vi "Edit Color List Dialog.vi"(10 "Color List":u32[](array[colorbox])=[16777225, 16448250, 16448250, 16448250, 16448250, 16448250, 16448250, 16448250, 16448250, 16448250], 11 "Color List Name":string) -> (0 "OK?":bool, 2 "Color List (out)":u32[](array[colorbox]), 3 "Color List Name (out)":string)   [LabVIEW 2021, in "Graphs.lvlib"]
uses:
  Graphs.lvlib
panel:
  in  "Cancel":bool
  in  "OK":bool
  out "# Colors":i32
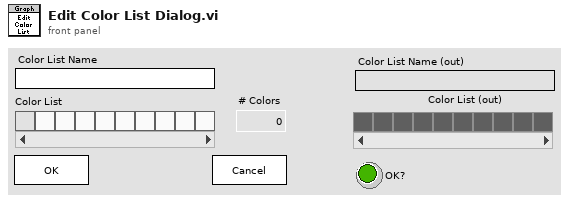
[diagram p1: front panel]
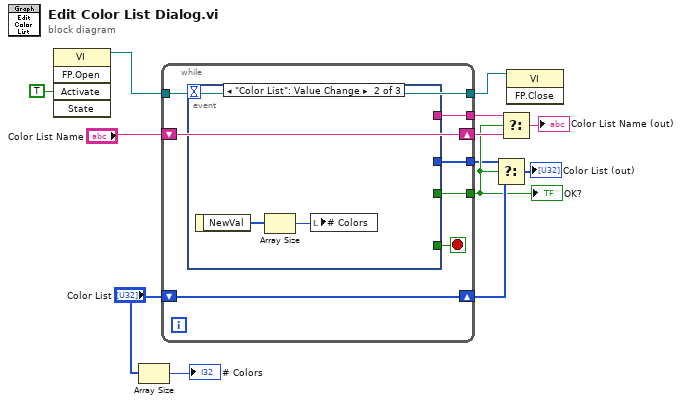
[diagram p0: block diagram]
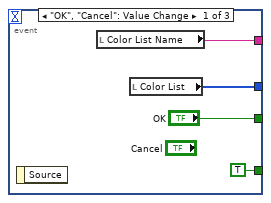
[diagram p2: hidden frame]
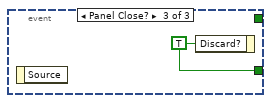
[diagram p3: hidden frame]
diagram:
  n1 = invoke class="VI" method="FP.Open"("Activate"=TRUE ("Activate?")) -> (reference out=w8:refnum<vi>)  [unwired: 4 in, 4 out]
  n2 = Array Size(array="Color List") -> (size(s)=→"# Colors":i32)
  n3 = while {
    tunnel: [w19] -> w3
    tunnel: w8 -> [w18]
    tunnel: [w18] -> w13
    shift-right: [w17] -> w12
    shift-left: "Color List" -> [w17]
    shift-right: [w16] -> w5
    shift-left: "Color List Name" -> [w16]
    tunnel: [w15] -> w2
    tunnel: [w14] -> w1
    stop <- w20 stop-if-true
    n4 = event shown="[1] \"Color List\": Value Change" {
      selector: _ -> [_ _ _]
      dyn-events: _ -> [_ _ _]
      timeout: _ -> [_ _ _]
      tunnel: [TRUE ("Discard?") _ w27] -> w20
      tunnel: ["OK" _ _] -> w19
      tunnel: [w22 _ _] -> w15
      tunnel: [w21 _ _] -> w14
      event "OK", "Cancel": Value Change {
        n5 = event-data() -> ()  [unwired: 1 in, 1 out]
        n6 = local read "Color List Name"() -> (w21:string)
        n7 = local read "Color List"() -> (w22:u32[])
      }
      event "Color List": Value Change {
        n8 = event-data() -> ("NewVal"=w26:u32[])  [unwired: 1 in]
        n9 = Array Size(array=w26) -> (size(s)=w25:i32)
        n10 = local write "# Colors"(w25) -> ()
      }
      event Panel Close? {
        w27 = TRUE ("Discard?")
        n11 = event-data() -> ()  [unwired: 1 in, 1 out]
        n12 = event-data("Discard?"=w27) -> ()  [unwired: 1 in, 1 out]
      }
    }
  }
  "OK?" <- w3
  n13 = Select(t=w2, s=w3, f=w12) -> (s? t:f=→"Color List (out)":u32[])
  n14 = Select(t=w1, s=w3, f=w5) -> (s? t:f=→"Color List Name (out)":string)
  n15 = invoke class="VI" method="FP.Close"(reference=w13) -> ()  [unwired: 2 in, 3 out]
